vi "LCDDrawLine.vi"(5 "y2":i32, 7 "x2":i32, 8 "error in (no error)":errorcluster, 9 "y1":i32, 10 "x1":i32, 11 "Device In":u64) -> (0 "error out":errorcluster, 3 "Device Out":u64)   [LabVIEW 2012, in "Phidget LCD.lvlib"]
doc: "${DrawLine:Header}"
uses:
  <instrlib>/Phidgets/Phidget LCD/Phidget LCD.lvlib
  <instrlib>/Phidgets/Phidget Common/Phidget Common.lvlib
  phidget22.dll
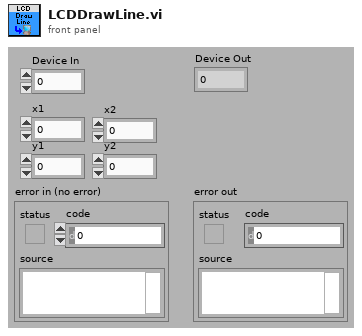
[diagram p1: front panel]
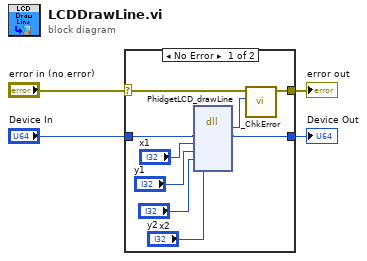
[diagram p0: block diagram]
diagram:
  n1 = case shown="No Error" "error in (no error)" {
    selector: "error in (no error)" -> [w13 w15]
    tunnel: [w12 w15] -> w3
    tunnel: "Device In" -> [w11 w14]
    tunnel: [w10 w14] -> w1
    frame No Error {
      n2 = dll-call lib="phidget22.*" fn="PhidgetLCD_drawLine"("phid"=w11, "x1"="x1", "y1"="y1", "x2"="x2", "y2"="y2") -> ("return type"=w9:i32, "phid"=w10:u64)  [unwired: 7 in, 2 out]
      n3 = call <instrlib>:"_ChkError.vi"("Return Code"=w9, "error in (no error)"=w13) -> ("error out"=w12:errorcluster)  [unwired: 9 in]
    }
    frame Error {
    }
  }
  "error out" <- w3
  "Device Out" <- w1
